vi "Read Configuration.vi"(8 "error in (no error)":errorcluster, 11 "Sensor General Class in":refnum<class "Sensor General Class.lvclass">) -> (0 "error out":errorcluster, 2 "Configuration":T1(array[cluster]), 3 "Sensor General Class out":refnum<class "Sensor General Class.lvclass">)   [LabVIEW 2020, in "Sensor General Class.lvclass"]
uses:
  Sensor General Class.lvclass
  Sensor General Class.lvclass/Sensor General Class.ctl
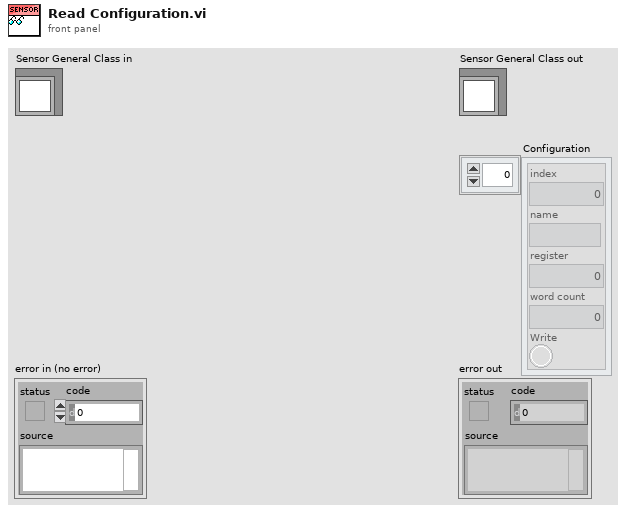
[diagram p1: front panel]
types:
  T1 = cluster{"index":i32, "name":string, "register":u16, "word count":u16, "Write":bool}[]
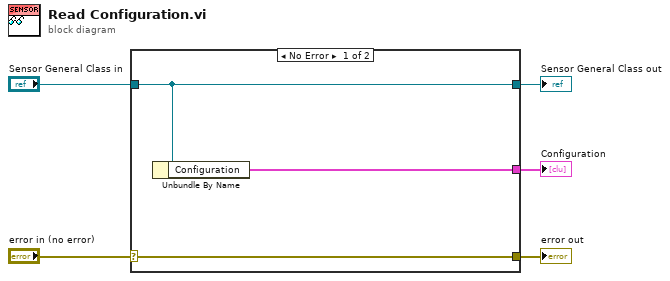
[diagram p0: block diagram]
diagram:
  n1 = case shown="No Error" "error in (no error)" {
    selector: "error in (no error)" -> [w8 w9]
    tunnel: [w8 w9] -> w4
    tunnel: [w7 w10] -> w2
    tunnel: "Sensor General Class in" -> [w7 w10]
    tunnel: [w6 _] -> w1
    frame No Error {
      n2 = Unbundle By Name(w7) -> ("Configuration"=w6:T1)
    }
    frame Error {
    }
  }
  "error out" <- w4
  "Sensor General Class out" <- w2
  "Configuration" <- w1
